vi "Assert BrowerIterator.vi"() -> ()   [LabVIEW 2015]
uses:
  BrowerComponent/BrowerComposite/BrowerComposite.lvclass
  BrowerComponent/BrowerLeaf/BrowerLeaf.lvclass
  Interface/Iterator.lvclass
  BrowerComponent/BrowerComponent/BrowerComponent.lvclass
panel:
  out "ComponentName 4":string
  out "ComponentName 3":string
  out "x = y?":bool
  out "HasNext?(True) 2":bool
  out "ComponentName 2":string
  out "ComponentName":string
  out "HasNext?(True)":bool
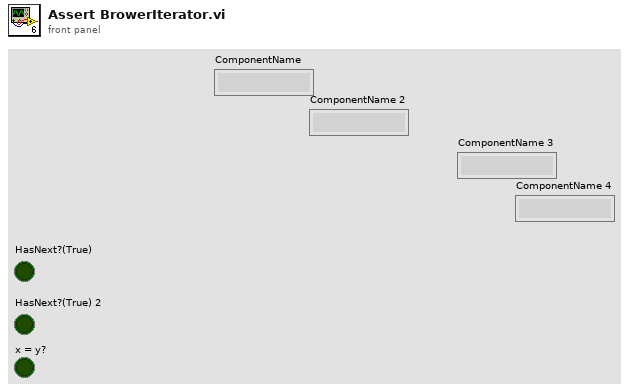
[diagram p1: front panel]
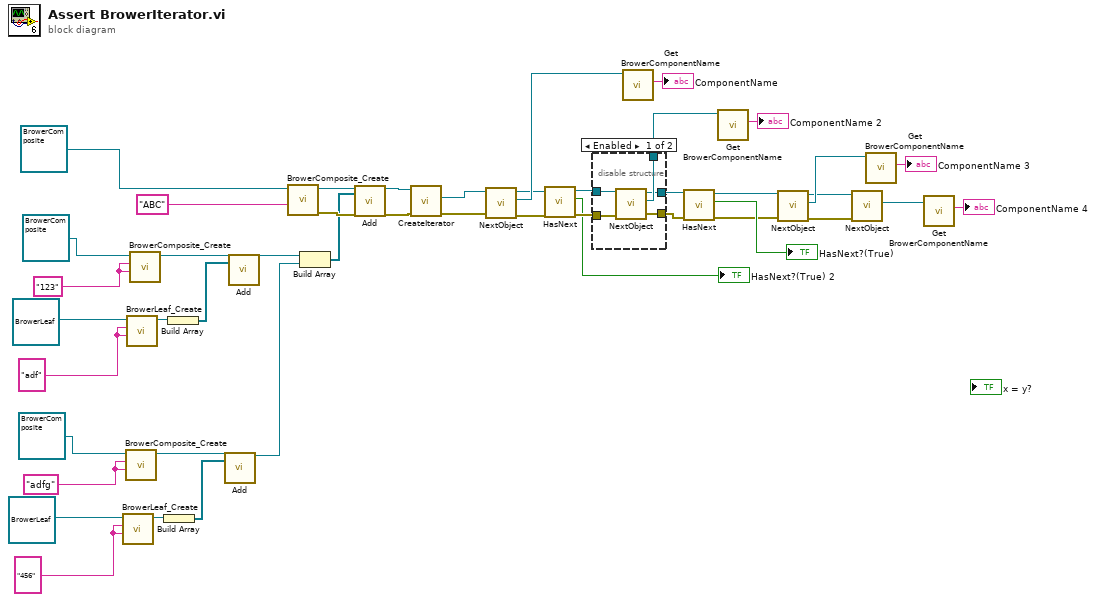
[diagram p0: block diagram]
diagram:
  w15 = "456" ("ComponentID")
  w14 = "adfg" ("ComponentName")
  w32 = "adf" ("ComponentID")
  w33 = "123" ("ComponentName")
  n1 = call "BrowerLeaf_Create.vi"("ComponentName"=w15, "ComponentID"=w15, "reference in"=refnum<class "BrowerLeaf.lvclass"> refnum ("BrowerLeaf")) -> ("reference out"=w13:refnum<class "BrowerLeaf.lvclass">)  [unwired: 7 in, 1 out]
  n2 = call "BrowerComposite_Create.vi"("ComponentName"=w14, "ComponentID"=w14, "reference in"=refnum<class "BrowerComposite.lvclass"> refnum ("BrowerComposite")) -> ("reference out"=w12:refnum<class "BrowerComposite.lvclass">)  [unwired: 7 in, 1 out]
  n3 = call "BrowerLeaf_Create.vi"("ComponentName"=w32, "ComponentID"=w32, "reference in"=refnum<class "BrowerLeaf.lvclass"> refnum ("BrowerLeaf")) -> ("reference out"=w35:refnum<class "BrowerLeaf.lvclass">)  [unwired: 7 in, 1 out]
  n4 = call "BrowerComposite_Create.vi"("ComponentName"=w33, "ComponentID"=w33, "reference in"=refnum<class "BrowerComposite.lvclass"> refnum ("BrowerComposite")) -> ("reference out"=w36:refnum<class "BrowerComposite.lvclass">)  [unwired: 7 in, 1 out]
  n5 = Build Array(w13) -> (w16:refnum<class "BrowerLeaf.lvclass">[])
  n6 = Build Array(w35) -> (w17:refnum<class "BrowerLeaf.lvclass">[])
  n7 = call-dynamic "Add.vi"("reference in"=w12, "BrowerComponents"=w16) -> ("reference out"=w9:refnum<class "BrowerComposite.lvclass">)  [unwired: 16 in, 1 out]
  n8 = call-dynamic "Add.vi"("reference in"=w36, "BrowerComponents"=w17) -> ("reference out"=w34:refnum<class "BrowerComposite.lvclass">)  [unwired: 16 in, 1 out]
  n9 = call "BrowerComposite_Create.vi"("ComponentName"="ABC", "reference in"=refnum<class "BrowerComposite.lvclass"> refnum ("BrowerComposite")) -> ("error out"=w42:errorcluster, "reference out"=w41:refnum<class "BrowerComposite.lvclass">)  [unwired: 8 in]
  n10 = Build Array(w34, w9) -> (w39:refnum<class "BrowerComposite.lvclass">[])
  n11 = call-dynamic "Add.vi"("reference in"=w41, "BrowerComponents"=w39, "error in (no error)"=w42) -> ("reference out"=w45:refnum<class "BrowerComposite.lvclass">, "error out"=w44:errorcluster)  [unwired: 15 in]
  n12 = call-dynamic "CreateIterator.vi"("error in (no error)"=w44, "BrowerComposite in"=w45) -> ("error out"=w28:errorcluster, "Iterator"=w29:refnum<class "Iterator.lvclass">)  [unwired: 7 in, 1 out]
  n13 = call-dynamic "NextObject.vi"("error in (no error)"=w28, "Iterator"=w29) -> ("error out"=w22:errorcluster, "BrowerComponent"=w27:refnum<class "BrowerComponent.lvclass">, "Iterator out"=w21:refnum<class "Iterator.lvclass">)  [unwired: 7 in]
  n14 = call-dynamic "HasNext.vi"("error in (no error)"=w22, "Iterator"=w21) -> ("error out"=w19:errorcluster, "HasNext?(False)"=→"HasNext?(True) 2":bool, "Iterator out"=w20:refnum<class "Iterator.lvclass">)  [unwired: 7 in]
  n15 = disable-structure shown="Enabled" {
    disable-tunnel: w19 -> [w50 w51]
    disable-tunnel: [w47 w51] -> w24
    disable-tunnel: w20 -> [w49 _]
    disable-tunnel: [w48 _] -> w26
    disable-tunnel: [w46 _] -> w25
    frame Enabled {
      n16 = call-dynamic "NextObject.vi"("error in (no error)"=w50, "Iterator"=w49) -> ("error out"=w47:errorcluster, "BrowerComponent"=w48:refnum<class "BrowerComponent.lvclass">, "Iterator out"=w46:refnum<class "Iterator.lvclass">)  [unwired: 7 in]
    }
    frame Disabled {
    }
  }
  n17 = call "Get BrowerComponentName.vi"("BrowerComponent in"=w27) -> ("ComponentName"=→"ComponentName":string)  [unwired: 8 in, 2 out]
  n18 = call-dynamic "HasNext.vi"("error in (no error)"=w24, "Iterator"=w25) -> ("error out"=w8:errorcluster, "HasNext?(False)"=→"HasNext?(True)":bool, "Iterator out"=w7:refnum<class "Iterator.lvclass">)  [unwired: 7 in]
  n19 = call "Get BrowerComponentName.vi"("BrowerComponent in"=w26) -> ("ComponentName"=→"ComponentName 2":string)  [unwired: 8 in, 2 out]
  n20 = call-dynamic "NextObject.vi"("error in (no error)"=w8, "Iterator"=w7) -> ("error out"=w3:errorcluster, "BrowerComponent"=w5:refnum<class "BrowerComponent.lvclass">, "Iterator out"=w4:refnum<class "Iterator.lvclass">)  [unwired: 7 in]
  n21 = call-dynamic "NextObject.vi"("error in (no error)"=w3, "Iterator"=w4) -> ("BrowerComponent"=w1:refnum<class "BrowerComponent.lvclass">)  [unwired: 7 in, 2 out]
  n22 = call "Get BrowerComponentName.vi"("BrowerComponent in"=w5) -> ("ComponentName"=→"ComponentName 3":string)  [unwired: 8 in, 2 out]
  n23 = call "Get BrowerComponentName.vi"("BrowerComponent in"=w1) -> ("ComponentName"=→"ComponentName 4":string)  [unwired: 8 in, 2 out]
